vi "player-coin.vi"(8 "error in (no error)":errorcluster, 9 "Game Road Numeric":i32, 10 "Game Coin Numeric":i32, 11 "Cluster":refnum<vi>) -> (0 "error out":errorcluster, 2 "Game Coin Ref":refnum<vi>, 3 "Game Road Ref":refnum<vi>)   [LabVIEW 2010]
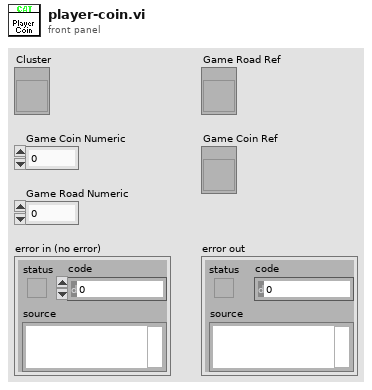
[diagram p1: front panel]
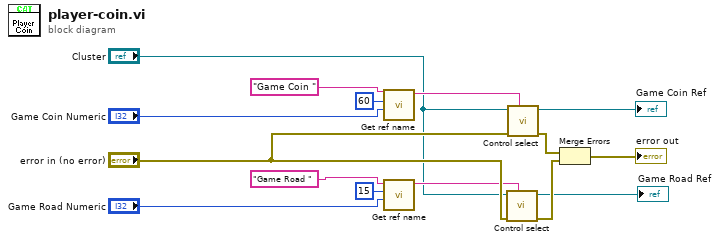
[diagram p0: block diagram]
diagram:
  n1 = call "Get ref name.vi"("i"="Game Coin Numeric", "step"=60, "name"="Game Coin ") -> ("resources"=w6:string)  [unwired: 8 in]
  n2 = call "Get ref name.vi"("i"="Game Road Numeric", "step"=15, "name"="Game Road ") -> ("resources"=w7:string)  [unwired: 8 in]
  n3 = call "Control select.vi"("resousce name"=w7, "error in (no error)"="error in (no error)", "Clust Refnum"="Cluster") -> ("error out"=w13:errorcluster, "Control Refnum"=→"Game Road Ref":refnum<vi>)  [unwired: 7 in]
  n4 = call "Control select.vi"("resousce name"=w6, "error in (no error)"="error in (no error)", "Clust Refnum"="Cluster") -> ("error out"=w14:errorcluster, "Control Refnum"=→"Game Coin Ref":refnum<vi>)  [unwired: 7 in]
  n5 = Merge Errors(w14, w13) -> (→"error out":errorcluster)
